vi "Line Follower.vi"(11 "speed":dbl) -> ()   [LabVIEW 2018]
uses:
  <vilib>/myRIO/Instrument Drivers/Onboard IO/AI/typedefs/AI Reference.ctl
  <vilib>/myRIO/Common/Instrument Driver Framework/Utilities/typedefs/myRIO Generic Hardware Reference.ctl
  <vilib>/myRIO/Common/Instrument Driver Framework/Utilities/typedefs/Hardware Version Enum.ctl
  <vilib>/myRIO/Common/Instrument Driver Framework/Utilities/typedefs/myRIO v1.0 Reference.ctl
  <vilib>/myRIO/Common/Instrument Driver Framework/Utilities/typedefs/Generic FPGA Reference.ctl
  <vilib>/myRIO/Common/Instrument Driver Framework/myRIO v1.0/AI/typedefs/AI Channels List.ctl
  <vilib>/myRIO/Common/Instrument Driver Framework/myRIO v1.0/AI/typedefs/AI Channels Enum.ctl
  <vilib>/myRIO/Common/Instrument Driver Framework/Utilities/typedefs/Analog Scaling Constants List.ctl
  <vilib>/myRIO/Common/Instrument Driver Framework/Utilities/typedefs/Analog Scaling Constants.ctl
  <vilib>/userdefined/High Color/nirio_resource_hc.ctl
  <vilib>/myRIO/Instrument Drivers/Onboard IO/DIO/typedefs/DIO Reference.ctl
  <vilib>/myRIO/Common/Instrument Driver Framework/myRIO v1.0/DIO/typedefs/DIO Channels List.ctl
  <vilib>/myRIO/Common/Instrument Driver Framework/myRIO v1.0/DIO/typedefs/DIO Channels Enum.ctl
  <vilib>/myRIO/Common/Instrument Driver Framework/Utilities/vis/Is FPGA Ref Available.vi
  <vilib>/myRIO/Common/Instrument Driver Framework/myRIO v1.0/AI/vis/myRIO v1.1 Open AI.vi
  <vilib>/myRIO/Instrument Drivers/Onboard IO/AI/vis/Read.vi
  <vilib>/myRIO/Common/Instrument Driver Framework/myRIO v1.0/DIO/vis/myRIO v1.1 Open DIO.vi
  <vilib>/myRIO/Instrument Drivers/Onboard IO/DIO/vis/Read.vi
  <vilib>/myRIO/Common/Instrument Driver Framework/Utilities/vis/Validate Channels.vi
  <vilib>/myRIO/Common/Instrument Driver Framework/myRIO v1.0/AI/vis/myRIO v1.0 Reserve AI.vi
  <vilib>/myRIO/Common/Instrument Driver Framework/myRIO v1.0/DIO/vis/myRIO v1.0 Reserve DIO.vi
  <vilib>/myRIO/Common/Instrument Driver Framework/myRIO v1.0/AI/vis/myRIO v1.0 Build MUX Configuration AI.vi
  <vilib>/myRIO/Common/Instrument Driver Framework/myRIO v1.0/Resource Manager/vis/myRIO v1.0 Reserve Channel List.vi
  <vilib>/myRIO/Common/Instrument Driver Framework/myRIO v1.0/DIO/vis/myRIO v1.0 Build MUX Configuration DIO.vi
  <vilib>/myRIO/Common/Instrument Driver Framework/myRIO v1.0/Resource Manager/vis/myRIO v1.0 Reserve Channel.vi
  <vilib>/myRIO/Common/Instrument Driver Framework/myRIO v1.0/Resource Manager/vis/myRIO v1.0 Unreserve Channel.vi
  <vilib>/myRIO/Common/Instrument Driver Framework/myRIO v1.0/Resource Manager/vis/myRIO v1.0 Create Configuration List.vi
  <vilib>/myRIO/Common/Instrument Driver Framework/myRIO v1.0/Resource Manager/vis/myRIO v1.0 Build Mutex Name.vi
  <vilib>/Utility/VariantDataType/GetNumericInfo.vi
  <vilib>/Utility/error.llb/Error Cluster From Error Code.vi
  <vilib>/myRIO/Common/Instrument Driver Framework/myRIO v1.0/myRIO v1.1 Open.vi
  <vilib>/myRIO/Common/Instrument Driver Framework/myRIO v1.0/AI/vis/myRIO v1.0 Get Scaling Constants AI.vi
  <vilib>/myRIO/Common/Instrument Driver Framework/Utilities/vis/IO Manager.vi
  <vilib>/myRIO/Common/Instrument Driver Framework/Utilities/vis/Configuration Manager.vi
  <vilib>/myRIO/Common/Instrument Driver Framework/myRIO v1.0/myRIO v1.0 Close.vi
  <vilib>/myRIO/Common/Instrument Driver Framework/myRIO v1.0/AI/vis/myRIO v1.0 Read AI.vi
  <vilib>/myRIO/Common/Instrument Driver Framework/myRIO v1.0/Resource Manager/vis/myRIO v1.0 Configure IO.vi
  <vilib>/myRIO/Common/Instrument Driver Framework/myRIO v1.0/DIO/vis/myRIO v1.0 Read DIO.vi
  <vilib>/myRIO/Express VI/Onboard IO/AI/AI Express VI.xnode
  <vilib>/myRIO/Instrument Drivers/Onboard IO/AI/vis/myRIO AI Open.xnode
  <vilib>/myRIO/Express VI/Onboard IO/DI/DI Express VI.xnode
  <vilib>/myRIO/Instrument Drivers/Onboard IO/DIO/vis/myRIO DIO Open.xnode
  <vilib>/myRIO/Instrument Drivers/Onboard IO/AI/AI.lvlib
  <vilib>/myRIO/Instrument Drivers/Onboard IO/DIO/DIO.lvlib
panel:
  in  "stop":bool
  out "back right":i16
  out "back left":i16
  out "front right":i16
  out "front left":i16
  out "right read":dbl
  out "left read":dbl
  in  "U":dbl
  in  "integral":dbl
  in  "last error":dbl
  in  "error":dbl
  in  "D":dbl
  in  "P":dbl
  in  "I":dbl
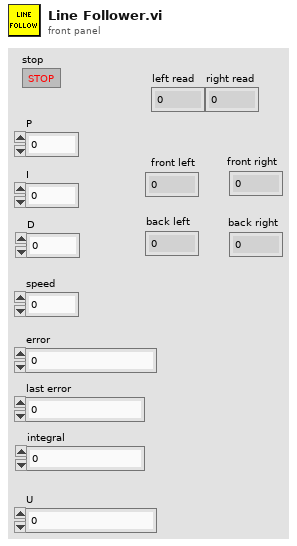
[diagram p1: front panel]
types:
  T1 = typedef "AI.lvlib/AI Reference.ctl" = cluster{"myRIO Reference":T2, "AI Channels List":T6, "AI Scaling Constants List":T8}
  T2 = typedef "myRIO Generic Hardware Reference.ctl" = cluster{"myRIO Model":T3, "myRIO Hardware Reference":T4}
  T3 = typedef "Hardware Version Enum.ctl" = enum16{"Unknown", "myRIO-1900", "myRIO-1950", "roboRIO", "NI ELVIS RIO CM", "ELVIS III"}
  T4 = typedef "myRIO v1.0 Reference.ctl" = cluster{"Generic FPGA Reference":T5, "Allow multiple opens":bool}
  T5 = typedef "Generic FPGA Reference.ctl" = refnum<k20>
  T6 = typedef "AI Channels List.ctl" = T7[]
  T7 = typedef "AI Channels Enum.ctl" = enum16{"Not Connected", "AudioIn/Left", "AudioIn/Right", "C/AI0", "C/AI1", "A/AI0", "A/AI1", "A/AI2", "A/AI3", "A/AI4", "A/AI5", "A/AI6", "A/AI7", "B/AI0", "B/AI1", "B/AI2", "B/AI3", "B/AI4", "B/AI5", "B/AI6", "B/AI7", "AI/AI0", "AI/AI1", "AI/AI2", "AI/AI3", "A/AI0 (DIFF)", "A/AI1 (DIFF)", "A/AI2 (DIFF)", "A/AI3 (DIFF)", "B/AI0 (DIFF)", "B/AI1 (DIFF)", "B/AI2 (DIFF)", "B/AI3 (DIFF)"}
  T8 = typedef "Analog Scaling Constants List.ctl" = T9[]
  T9 = typedef "Analog Scaling Constants.ctl" = cluster{"LSB Weight (Volts)":dbl, "Offset (Volts)":dbl, "Signed?":bool}
  T10 = typedef "nirio_resource_hc.ctl" = tag
  T11 = typedef "DIO.lvlib/DIO Reference.ctl" = cluster{"myRIO Reference":T2, "DIO Channels List":T12}
  T12 = typedef "DIO Channels List.ctl" = T13[]
  T13 = typedef "DIO Channels Enum.ctl" = enum16{"Not Connected", "C/DIO0", "C/DIO1", "C/DIO2", "C/DIO3", "C/DIO4", "C/DIO5", "C/DIO6", "C/DIO7", "A/DIO0", "A/DIO1", "A/DIO2", "A/DIO3", "A/DIO4", "A/DIO5", "A/DIO6", "A/DIO7", "A/DIO8", "A/DIO9", "A/DIO10", "A/DIO11", "A/DIO12", "A/DIO13", "A/DIO14", "A/DIO15", "A/DIO16", "A/DIO17", "A/DIO18", "A/DIO19", "B/DIO0", "B/DIO1", "B/DIO2", "B/DIO3", "B/DIO4", "B/DIO5", "B/DIO6", "B/DIO7", "B/DIO8", "B/DIO9", "B/DIO10", "B/DIO11", "B/DIO12", "B/DIO13", "B/DIO14", "B/DIO15", "B/DIO16", "B/DIO17", "B/DIO18", "B/DIO19", "LED0", "LED1", "LED2", "LED3", "Button0", "DIO/DIO0", "DIO/DIO1", "DIO/DIO2", "DIO/DIO3", "DIO/DIO4", "DIO/DIO5", "DIO/DIO6", "DIO/DIO7", "DIO/DIO8", "DIO/DIO9", "SPI/CS0", "SPI/CS1", "SPI/CS2", "SPI/CS3", "LED RADIO (Green)", "LED RADIO (Red)", "LED COMM (Green)", "LED COMM (Red)", "LED MODE (Green)", "LED MODE (Red)"}
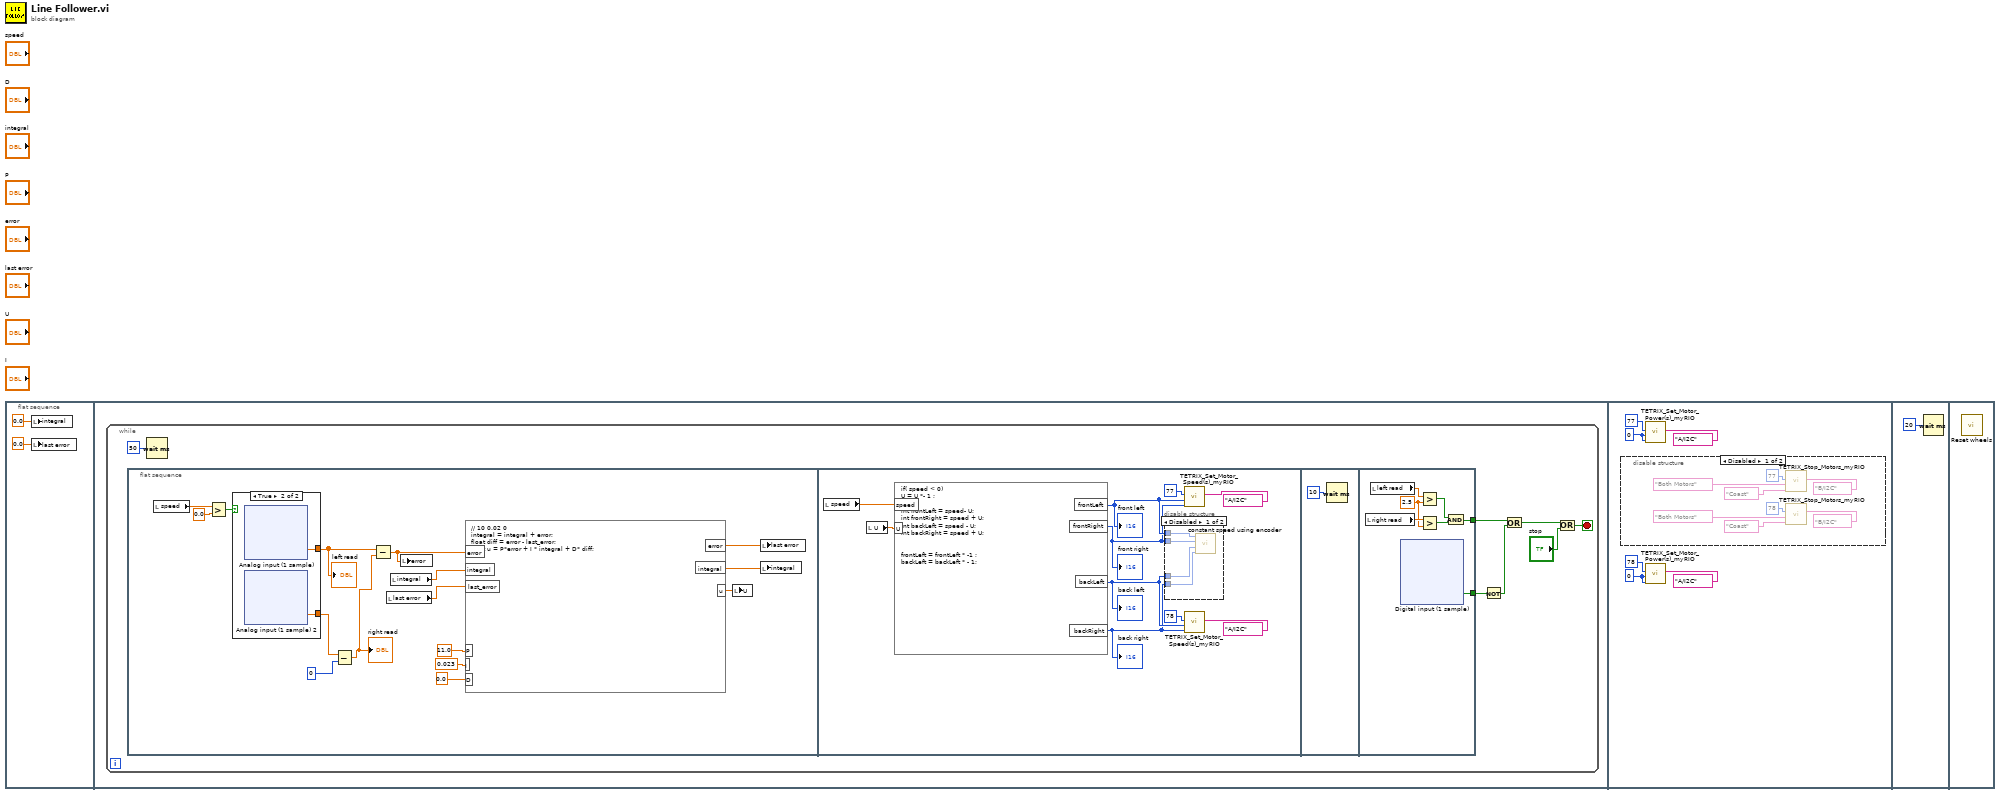
[diagram p0: block diagram]
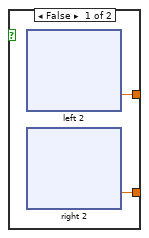
[diagram p2: hidden frame]
diagram:
  n1 = flat-sequence {
    frame #0 {
      n2 = local write "integral"(0.0 ("integral")) -> ()
      n3 = local write "last error"(0.0 ("last error")) -> ()
    }
    frame #1 {
      n4 = while {
        stop <- w8 stop-if-true
        n5 = flat-sequence {
          tunnel: [w194] -> w7
          tunnel: [w193] -> w5
          frame #0 {
            n6 = local read "speed"() -> (w15:dbl)
            n7 = Greater?(x=w15, y=0.0) -> (0:w14:bool)
            n8 = case shown="True" w14 {
              tunnel: [w26 w103] -> w12
              tunnel: [w27 w102] -> w16
              frame False {
                n9 = xnode "left 2"() -> ("A/AI2 (Pin 7)"=w27:dbl)  [unwired: 1 in, 1 out]
                n10 = xnode "right 2"() -> ("A/AI3 (Pin 9)"=w26:dbl)  [unwired: 1 in, 1 out]
              }
              frame True {
                n11 = xnode "Analog input (1 sample)"() -> ("A/AI1 (Pin 5)"=w102:dbl)  [unwired: 1 in, 1 out]
                n12 = xnode "Analog input (1 sample) 2"() -> ("A/AI0 (Pin 3)"=w103:dbl)  [unwired: 1 in, 1 out]
              }
            }
            "left read" <- w16
            n13 = Subtract(x=w12, y=0) -> (x-y=w10:dbl)
            "right read" <- w10
            n14 = Subtract(x=w16, y=w10) -> (x-y=w22:dbl)
            n15 = local read "last error"() -> (w20:dbl)
            n16 = local read "integral"() -> (w21:dbl)
            n17 = local write "error"(w22) -> ()
            n18 = formula code="// 10 0.02 0\nintegral = integral + error;\nfloat diff = error - last_error;\nfloat u = P*error + I * integral + D* diff;"("error"=w22, "integral"=w21, "last_error"=w20, "P"=11.0 ("input variable"), "I"=0.023 ("input variable"), "D"=0.0 ("input variable")) -> ("error"=w25:dbl, "integral"=w24:dbl, "u"=w23:dbl)
            n19 = local write "U"(w23) -> ()
            n20 = local write "last error"(w25) -> ()
            n21 = local write "integral"(w24) -> ()
          }
          frame #1 {
            n22 = local read "speed"() -> (w187:dbl)
            n23 = local read "U"() -> (w186:dbl)
            n24 = formula code="if( speed < 0)\nU = U *- 1 ;\n\nint frontLeft = speed- U;\nint frontRight = speed + U;\nint backLeft = speed - U;\nint backRight = speed + U;\n\n\nfrontLeft = frontLeft * -1 ;\nbackLeft = backLeft * - 1;"("speed"=w187, "U"=w186) -> ("frontLeft"=w185:i32, "frontRight"=w184:i32, "backLeft"=w183:i32, "backRight"=w182:i32)
            "front left" <- w185
            "front right" <- w184
            "back left" <- w183
            "back right" <- w182
            n25 = disable-structure shown="Disabled" {
              disable-tunnel: w185 -> [w191 _]
              disable-tunnel: w184 -> [w190 _]
              disable-tunnel: w183 -> [w189 _]
              disable-tunnel: w182 -> [w188 _]
              frame Disabled {
                n26 = call "constant speed using encoder.vi"("s78_2"=w188, "s78_1"=w189, "s77_2"=w190, "s77_1"=w191) -> ()  [unwired: 2 in]
              }
              frame Enabled {
              }
            }
            n27 = call <vilib>:"TETRIX_Set_Motor_Speed(s)_myRIO.vi"("myRIO MXP Port A/B"=tag "A/I2C", "Motor 2 Speed (Degrees per second). Sign (+/-)  sets direction."=w184, "Motor 1 Speed (Degrees per second). Sign (+/-)  sets direction."=w185, "Controller ID#  (I2C Address)"=u8 77) -> ()  [unwired: 3 in, 1 out]
            n28 = call <vilib>:"TETRIX_Set_Motor_Speed(s)_myRIO.vi"("myRIO MXP Port A/B"=tag "A/I2C", "Motor 2 Speed (Degrees per second). Sign (+/-)  sets direction."=w182, "Motor 1 Speed (Degrees per second). Sign (+/-)  sets direction."=w183, "Controller ID#  (I2C Address)"=u8 78) -> ()  [unwired: 3 in, 1 out]
          }
          frame #2 {
            n29 = Wait (ms)(milliseconds to wait=u32 10) -> ()  [unwired: 1 out]
          }
          frame #3 {
            w197 = 2.5 ("y")
            n30 = local read "right read"() -> (w198:dbl)
            n31 = local read "left read"() -> (w199:dbl)
            n32 = xnode "Digital input (1 sample)"() -> ("B/DIO0 (Pin 11)"=w193:bool)  [unwired: 1 in, 1 out]
            n33 = Greater?(x=w199, y=w197) -> (0:w196:bool)
            n34 = Greater?(x=w198, y=w197) -> (0:w195:bool)
            n35 = And(x=w196, y=w195) -> (x .and. y?=w194:bool)
          }
        }
        n36 = Wait (ms)(milliseconds to wait=u32 50) -> ()  [unwired: 1 out]
        n37 = Not(x=w5) -> (.not. x?=w4:bool)
        n38 = Or(x=w7, y=w4) -> (x .or. y?=w6:bool)
        n39 = Or(x=w6, y="stop") -> (x .or. y?=w8:bool)
      }
    }
    frame #2 {
      w235 = i8 0 ("Motor 1 Power (-100 to 100)  0 = Coast Stop  125 = Brake Stop")
      w238 = i8 0 ("Motor 1 Power (-100 to 100)  0 = Coast Stop  125 = Brake Stop")
      n40 = disable-structure shown="Disabled" {
        frame Disabled {
          n41 = call <vilib>:"TETRIX_Stop_Motors_myRIO.vi"("myRIO MXP Port A/B"=tag "B/I2C", "Stop Mode"="Coast", "Select Channel"="Both Motors", "Controller ID#  (I2C Address)"=u8 77) -> ()  [unwired: 3 in, 1 out]
          n42 = call <vilib>:"TETRIX_Stop_Motors_myRIO.vi"("myRIO MXP Port A/B"=tag "B/I2C", "Stop Mode"="Coast", "Select Channel"="Both Motors", "Controller ID#  (I2C Address)"=u8 78) -> ()  [unwired: 3 in, 1 out]
        }
        frame Enabled {
        }
      }
      n43 = call <vilib>:"TETRIX_Set_Motor_Power(s)_myRIO.vi"("myRIO MXP Port A/B"=tag "A/I2C", "Motor 2 Power (-100 to 100)  0 = Coast Stop  125 = Brake Stop"=w238, "Motor 1 Power (-100 to 100)  0 = Coast Stop  125 = Brake Stop"=w238, "Controller ID#  (I2C Address)"=u8 77) -> ()  [unwired: 3 in, 1 out]
      n44 = call <vilib>:"TETRIX_Set_Motor_Power(s)_myRIO.vi"("myRIO MXP Port A/B"=tag "A/I2C", "Motor 2 Power (-100 to 100)  0 = Coast Stop  125 = Brake Stop"=w235, "Motor 1 Power (-100 to 100)  0 = Coast Stop  125 = Brake Stop"=w235, "Controller ID#  (I2C Address)"=u8 78) -> ()  [unwired: 3 in, 1 out]
    }
    frame #3 {
      n45 = Wait (ms)(milliseconds to wait=u32 20) -> ()  [unwired: 1 out]
    }
    frame #4 {
      n46 = call "Reset wheels.vi"() -> ()  [unwired: 12 in]
    }
  }
